vi "SpecAn Configure Common.vi"(0 "RFmx Handle In":refnum<k21>, 1 "Selector String":string, 5 "Common Configuration":T1={"Center Frequency (Hz)"=1000000000.0, "Reference Level (dBm)"=0.0, "External Attenuation (dB)"=0.0, "Trigger Enabled"=TRUE, "Selected Ports"="", "IQ Power Edge Level (dB or dBm)"=0.0, "IQ Power Edge Source"="PXI_Trig0"} {"IQ Power Edge Level (dB or dBm)" format="%.2p"; "External Attenuation (dB)" format="%.2f"; "Reference Level (dBm)" format="%.2f"; "Center Frequency (Hz)" format="%.6p"}, 11 "error in (no error)":errorcluster) -> (4 "RFmx Handle Out":refnum<k21>, 15 "error out":errorcluster)   [LabVIEW 2019, in "RFmxSpecAn.lvlib"]
doc: "Configures common measurement settings for the personality."
uses:
  RFmxSpecAn.lvlib
  Common/SA Common Configuration.ctl
  <vilib>/RFmx/SpecAn/mx/RFmxSpecAn.llb/RFmxSpecAn Configure IQ Power Edge Trigger.vi
  <resource>/objmgr/RFmxSpecAn.rc
  Common/Common.lvlib
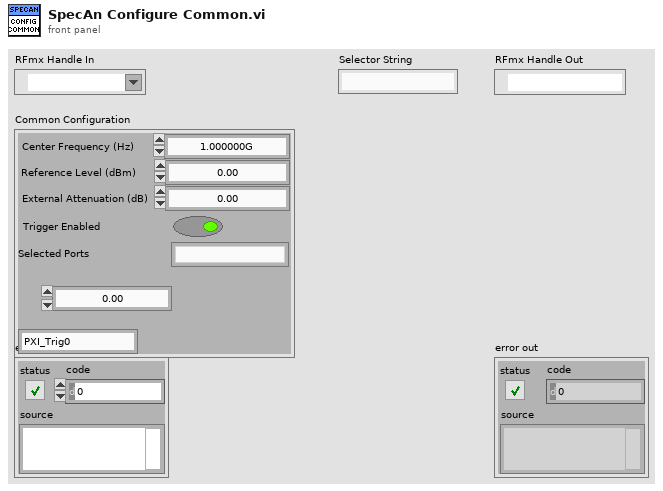
[diagram p1: front panel]
types:
  T1 = typedef "Common.lvlib/SA Common Configuration.ctl" = cluster{"Center Frequency (Hz)":dbl, "Reference Level (dBm)":dbl, "External Attenuation (dB)":dbl, "Trigger Enabled":bool, "Selected Ports":string, "IQ Power Edge Level (dB or dBm)":dbl, "IQ Power Edge Source":string}
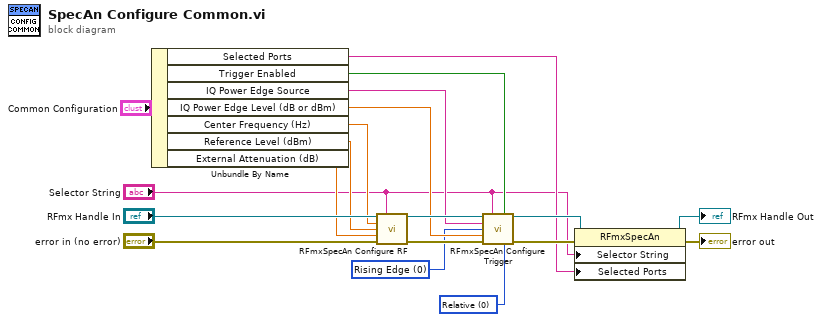
[diagram p0: block diagram]
diagram:
  w1 = 0 items=["Relative", "Absolute"] ("IQ Power Edge Level Type")
  w5 = 0 items=["Rising Edge", "Falling Edge"] ("Digital Edge")
  n1 = Unbundle By Name("Common Configuration") -> ("Selected Ports"=w4:string, "Trigger Enabled"=w9:bool, "IQ Power Edge Source"=w8:string, "IQ Power Edge Level (dB or dBm)"=w7:dbl, "Center Frequency (Hz)"=w15:dbl, "Reference Level (dBm)"=w14:dbl, "External Attenuation (dB)"=w13:dbl)
  n2 = call <vilib>:"RFmxSpecAn Configure RF.vi"("Instrument Handle In"="RFmx Handle In", "Selector String"="Selector String", "Center Frequency (Hz)"=w15, "Reference Level"=w14, "External Attenuation (dB)"=w13, "error in (no error)"="error in (no error)") -> ("Instrument Handle Out"=w19:refnum<k21>, "error out"=w18:errorcluster)  [unwired: 8 in]
  n3 = call-poly <vilib>:"RFmxSpecAn Configure Trigger.vi"("Instrument Handle In"=w19, "Selector String"="Selector String", "Enable Trigger?"=w9, "IQ Power Edge Source"=w8, "IQ Power Edge Slope"=w5, "IQ Power Edge Level (dB or dBm)"=w7, "error in (no error)"=w18, "IQ Power Edge Level Type"=w1) -> ("Instrument Handle Out"=w6:refnum<k21>, "error out"=w11:errorcluster)  [unwired: 6 in]
  n4 = property class="RFmxSpecAn"(reference=w6, error in=w11, "Selector String"="Selector String", "Selected Ports"=w4) -> (reference out=→"RFmx Handle Out":refnum<k21>, error out=→"error out":errorcluster)
